vi "gl_funct TIFF export globals.vi"() -> ()   [LabVIEW 2013]
uses:
  Typedefs/Funct TIFF exporter ctrl refs.ctl
  Typedefs/Exported TIFF type.ctl
panel:
  in  "Funct TIFF export-Window is open":bool
  in  "Funct TIFF export-Bring to front":bool
  in  "Funct TIFF exporter ctrl refs":T1
  in  "Stop TIFF export":bool
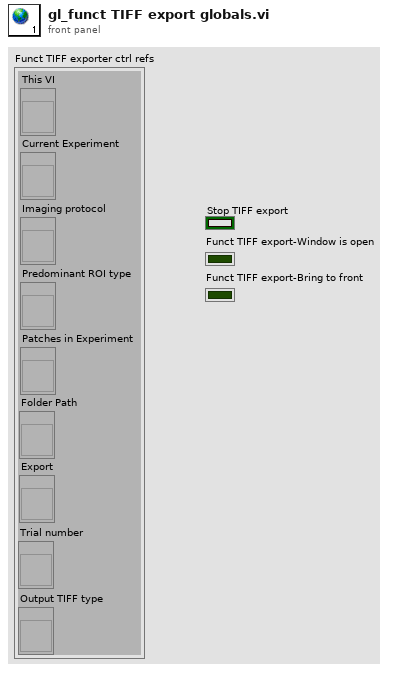
[diagram p1: front panel]
types:
  T1 = typedef "Funct TIFF exporter ctrl refs.ctl" = cluster{"This VI":refnum<vi>, "Current Experiment":refnum<vi>, "Imaging protocol":refnum<vi>, "Predominant ROI type":refnum<vi>, "Patches in Experiment":refnum<vi>, "Folder Path":refnum<vi>, "Export":refnum<vi>, "Trial number":refnum<vi>, "Output TIFF type":refnum<vi>}
diagram:
